vi "GetDataExplorerSpecificTdmsFileProperties.vi"(8 "error in (no error)":errorcluster) -> (0 "error out":errorcluster, 2 "TDMS properties":T1[](array[typedef]))   [LabVIEW 2017, in "Tdms.lvlib"]
doc: "Returns miscellaneous properties on which the Data Explorer software relies. Use this VI in processes that write TDMS files that users will load in the Data Explorer software. The property value is constant, so you do not need to set it."
uses:
  <vilib>/addons/InsightCM/Utilities/Tdms/Tdms.lvlib
  <vilib>/addons/InsightCM/Utilities/Tdms/controls/Property.ctl
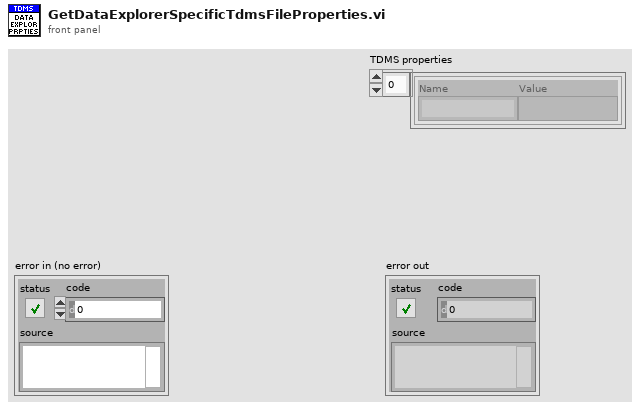
[diagram p1: front panel]
types:
  T1 = typedef "Tdms.lvlib/Property.ctl" = cluster{"Name":string, "Value":variant}
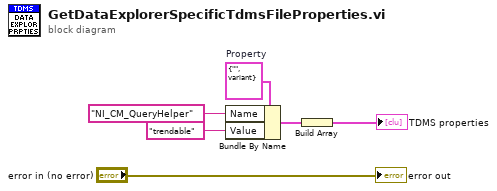
[diagram p0: block diagram]
diagram:
  w5 = T1 {"Name"="", "Value"=variant}  # Property
  n1 = Bundle By Name(cluster=w5, "Name"="NI_CM_QueryHelper", "Value"="trendable") -> (w4:T1)
  n2 = Build Array(w4) -> (→"TDMS properties":T1[])
  "error out" <- "error in (no error)"
